vi "Msg and Actor Init.vi"(9 "Type Name Library File Path":T1, 10 "Tree Ref":refnum<vi>) -> ()   [LabVIEW 2020, in "_Shared.lvlib" / "Tree.lvlib"]
uses:
  Tree.lvlib
  Type Name Library File Path.ctl
  Type.ctl
  Name Library File Path.ctl
  _Shared.lvlib
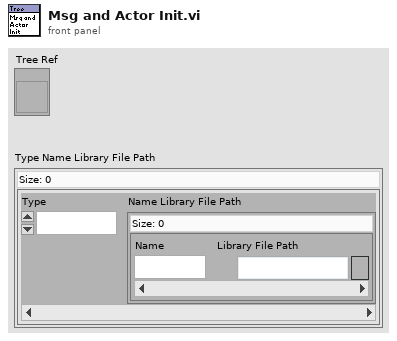
[diagram p1: front panel]
types:
  T1 = typedef "_Shared.lvlib/Type Name Library File Path.ctl" = map{T2, T3}
  T2 = typedef "_Shared.lvlib/Type.ctl" = enum16{"Actor", "Msg"}
  T3 = typedef "_Shared.lvlib/Name Library File Path.ctl" = map{string, path}
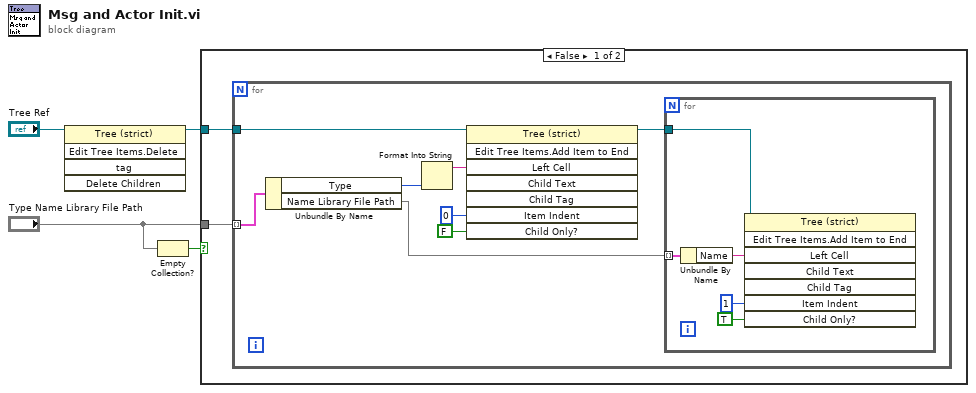
[diagram p0: block diagram]
diagram:
  n1 = invoke class="Tree (strict)" method="Edit Tree Items.Delete"(reference="Tree Ref") -> (reference out=w1:refnum<vi>)  [unwired: 4 in, 4 out]
  n2 = Empty Collection?(1:"Type Name Library File Path") -> (0:w3:bool)
  n3 = case shown="False" w3 {
    tunnel: "Type Name Library File Path" -> [w6 _]
    tunnel: w1 -> [w5 _]
    frame False {
      n4 = for {
        tunnel: w6 -> [w14] mode=indexing
        tunnel: w5 -> [w11]
        n5 = Unbundle By Name(w14) -> ("Type"=w13:T2, "Name Library File Path"=w9:T3)
        n6 = Format Into String(w13) -> (resulting string=w12:string)  [unwired: 3 in, 1 out]
        n7 = invoke class="Tree (strict)" method="Edit Tree Items.Add Item to End"(reference=w11, "Left Cell"=w12, "Item Indent"=0 ("New Item Indentation"), "Child Only?"=FALSE) -> (reference out=w10:refnum<vi>)  [unwired: 4 in, 7 out]
        n8 = for {
          tunnel: w10 -> [w19]
          tunnel: w9 -> [w18] mode=indexing
          n9 = Unbundle By Name(w18) -> ("Name"=w17:string)
          n10 = invoke class="Tree (strict)" method="Edit Tree Items.Add Item to End"(reference=w19, "Left Cell"=w17, "Item Indent"=1 ("New Item Indentation"), "Child Only?"=TRUE) -> ()  [unwired: 4 in, 8 out]
        }
      }
    }
    frame True {
    }
  }
